vi "Get Region.vi"(10 "x":i32, 11 "y":i32) -> (3 "region":string)   [LabVIEW 2021, in "d22.lvlib"]
uses:
  d22.lvlib
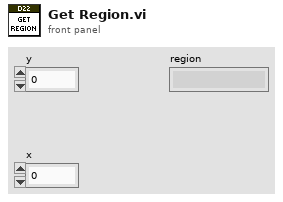
[diagram p1: front panel]
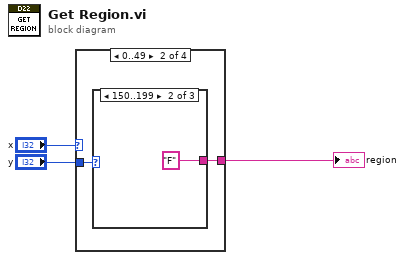
[diagram p0: block diagram]
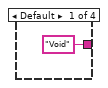
[diagram p2: hidden frame]
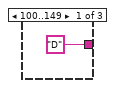
[diagram p3: hidden frame]
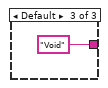
[diagram p4: hidden frame]
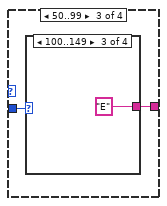
[diagram p5: hidden frame]
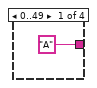
[diagram p6: hidden frame]
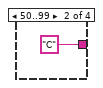
[diagram p7: hidden frame]
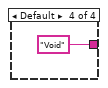
[diagram p8: hidden frame]
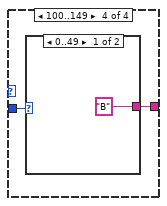
[diagram p9: hidden frame]
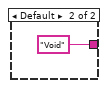
[diagram p10: hidden frame]
diagram:
  n1 = case shown="0..49" "x" {
    tunnel: "y" -> [_ w5 w10 w16]
    tunnel: ["Void" w6 w11 w17] -> w3
    frame Default {
    }
    frame 0..49 {
      n2 = case shown="150..199" w5 {
        tunnel: ["D" "F" "Void"] -> w6
        frame 100..149 {
        }
        frame 150..199 {
        }
        frame Default {
        }
      }
    }
    frame 50..99 {
      n3 = case shown="100..149" w10 {
        tunnel: ["A" "C" "E" "Void"] -> w11
        frame 0..49 {
        }
        frame 50..99 {
        }
        frame 100..149 {
        }
        frame Default {
        }
      }
    }
    frame 100..149 {
      n4 = case shown="0..49" w16 {
        tunnel: ["B" "Void"] -> w17
        frame 0..49 {
        }
        frame Default {
        }
      }
    }
  }
  "region" <- w3
